vi "qSWT.vi"(0 "System no.":i32=1 min=1 max=4 step=1, 2 "Axis":string, 4 "Index":i32=1 min=1 max=5 step=1, 5 "error in":errorcluster) -> (14 "Value":dbl, 19 "error out":errorcluster)   [LabVIEW 2026]
doc: "Returns wave table point with given index for given axis."
panel:
  # "Returns wave table point with given index for given axis."
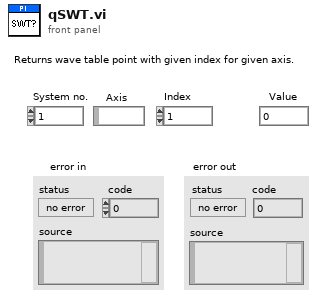
[diagram p1: front panel]
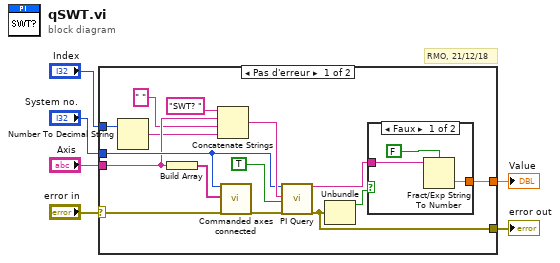
[diagram p0: block diagram]
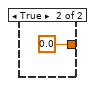
[diagram p2: hidden frame]
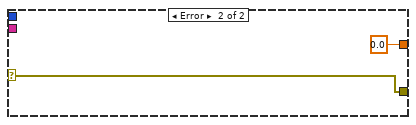
[diagram p3: hidden frame]
diagram:
  # "RMO, 21/12/18"
  n1 = case shown="Pas d'erreur" "error in" {
    selector: "error in" -> [w9 w26]
    tunnel: [w20 0.0] -> w6
    tunnel: [w8 w26] -> w5
    tunnel: "Index" -> [w10 _]
    tunnel: "System no." -> [w16 _]
    tunnel: "Axis" -> [w13 _]
    frame No Error {
      n2 = Number To Decimal String(number=w10) -> (decimal integer string=w11:string)  [unwired: 1 out]
      n3 = Build Array(w13) -> (w18:string[])
      n4 = Concatenate Strings("SWT? ", w13, " " ("string"), w11) -> (w17:string)
      n5 = call "Commanded axes connected.vi"("System no."=w16, "Commanded axes"=w18, "error in"=w9) -> ("error out"=w15:errorcluster)  [unwired: 1 in, 15 out]
      n6 = call "PI Query.vi"("System no."=w16, "String to send"=w17, "Attach termination char.?"=TRUE ("Attach Linefeed?"), "error in"=w15) -> ("String read"=w7:string, "error out"=w8:errorcluster)  [unwired: 3 in, 11 out]
      n7 = Unbundle(w8) -> ("status"=w21:bool)  [unwired: 2 out]
      n8 = case shown="Faux" w21 {
        tunnel: w7 -> [w23 _]
        tunnel: [w24 0.0] -> w20
        frame False {
          n9 = Fract/Exp String To Number(use system decimal point (T)=FALSE, string=w23) -> (number=w24:dbl)  [unwired: 3 out]
        }
        frame True {
        }
      }
    }
    frame Error {
    }
  }
  "error out" <- w5
  "Value" <- w6
